vi "TCP-IP Mgr.Show.vi"(8 "error in":errorcluster) -> (0 "error out":errorcluster)   [LabVIEW 2017, in "TCP-IP Mgr.lvlib"]
uses:
  TCP-IP Mgr.lvlib
  <vilib>/KATE/Module/Window/Window.Task, Action.ctl
  <vilib>/KATE/Module/Module Utils.lvlib
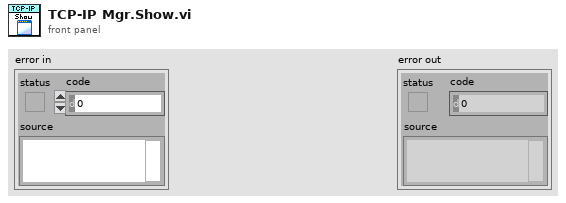
[diagram p1: front panel]
types:
  T1 = typedef "KATE_Lib.lvlib/Module Utils.lvlib/Window.Task, Action.ctl" = enum16{"Resize()", "Show Panel(Bool)", "Show Scroll Bars(Bool)", "Dock to SubPanel(SubPanel Ref)", "Undock from SubPanel()", "Return to SubPanel()", "Go To Maint Tab()", "Show Maint Tab(Bool)", "Open Block Diagram()"}
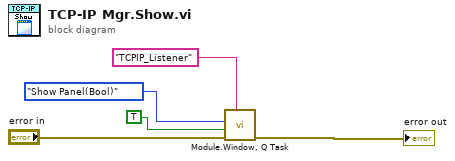
[diagram p0: block diagram]
diagram:
  n1 = call <vilib>:"Module.Window, Q Task.vi"("Q Name"="TCPIP_Listener" ("name (unnamed)"), "error in"="error in", "Show"=TRUE, "Action"=Window.Task,_Action."Show Panel(Bool)") -> ("error out"=→"error out":errorcluster)  [unwired: 6 in, 1 out]
